vi "-Send_And_Receive_Message.vi"(8 "error in (no error)":errorcluster, 10 "Message To Send":string, 11 "Postgres Connector In":refnum<class "Postgres Connector.lvclass">) -> (0 "error out":errorcluster, 2 "data out":string, 3 "Postgres Connector Out":refnum<class "Postgres Connector.lvclass">)   [LabVIEW 2019, in "PG_LIB.lvlib" / "Postgres Connector.lvclass"]
doc: "This send the message of the client to the Postgres database using TCP, then read the answer from the database."
uses:
  Postgres Connector.lvclass
  Postgres Connector.lvclass/Postgres Connector.ctl
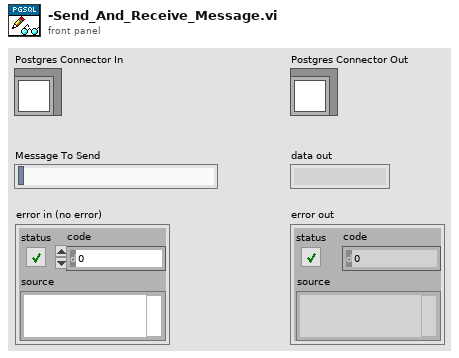
[diagram p1: front panel]
types:
  T1 = enum16{"Standard", "Buffered", "CRLF", "Immediate"}
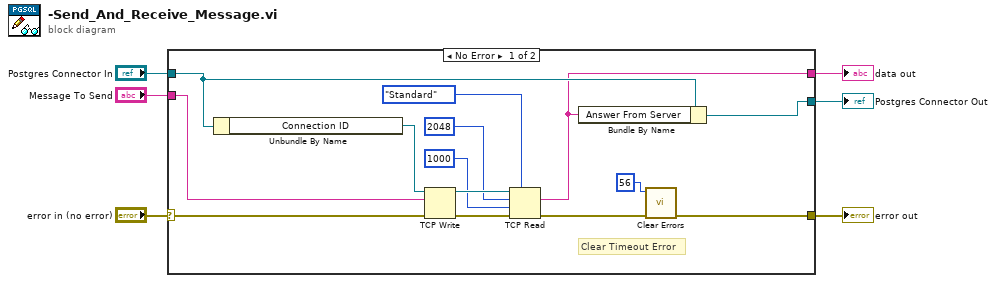
[diagram p0: block diagram]
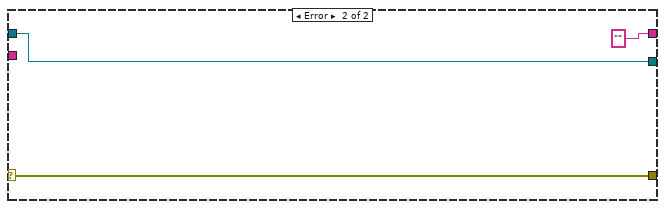
[diagram p2: hidden frame]
diagram:
  n1 = case shown="No Error" "error in (no error)" {
    selector: "error in (no error)" -> [w17 w23]
    tunnel: "Postgres Connector In" -> [w15 w22]
    tunnel: [w16 w23] -> w2
    tunnel: [w14 w22] -> w5
    tunnel: "Message To Send" -> [w18 _]
    tunnel: [w12 "" ("data out")] -> w1
    frame No Error {
      # "Clear Timeout Error"
      n2 = Unbundle By Name(w15) -> ("Connection ID"=w13:refnum<k5>)
      n3 = TCP Write(connection ID=w13, data in=w18, error in (no error)=w17) -> (connection ID out=w19:refnum<k5>, error out=w20:errorcluster)  [unwired: 1 in, 1 out]
      n4 = TCP Read(connection ID=w19, bytes to read=2048, error in (no error)=w20, 7:T1."Standard" ("mode (standard)"), 9:1000 ("timeout ms (25000)")) -> (data out=w12:string, error out=w11:errorcluster)  [unwired: 1 out]
      n5 = Bundle By Name(cluster=w15, "Answer From Server"=w12) -> (w14:refnum<class "Postgres Connector.lvclass">)
      n6 = call <vilib>:"Clear Errors.vi"("error in (no error)"=w11, "specific error code to clear (0: all)"=56) -> ("error out"=w16:errorcluster)  [unwired: 4 in, 1 out]
    }
    frame Error {
    }
  }
  "Postgres Connector Out" <- w5
  "error out" <- w2
  "data out" <- w1
